vi "ATEQread气密机一.vi"(7 "baud rate (9600)":u32=57600 caption="波特率(9600)", 8 "VISA resource name":refnum<visa-resource-name>="COM3" caption="COM", 9 "从站地址":u8=2 format="%x", 10 "Read Address":u16 format="%x", 11 "The number of Read":u32) -> (0 "Read Values":string, 1 "ReturnResultValues":u16[](array[numeric]), 2 "Read Status":bool)   [LabVIEW 2014]
uses:
  <vilib>/Instr/_visa.llb/VISA Configure Serial Port (Instr).vi
panel:
  out "Serial Settings:Number of Bytes at Serial Port":u32
  out "Result":string
  out "Read Return Value":string
  out "Send Read Date":string
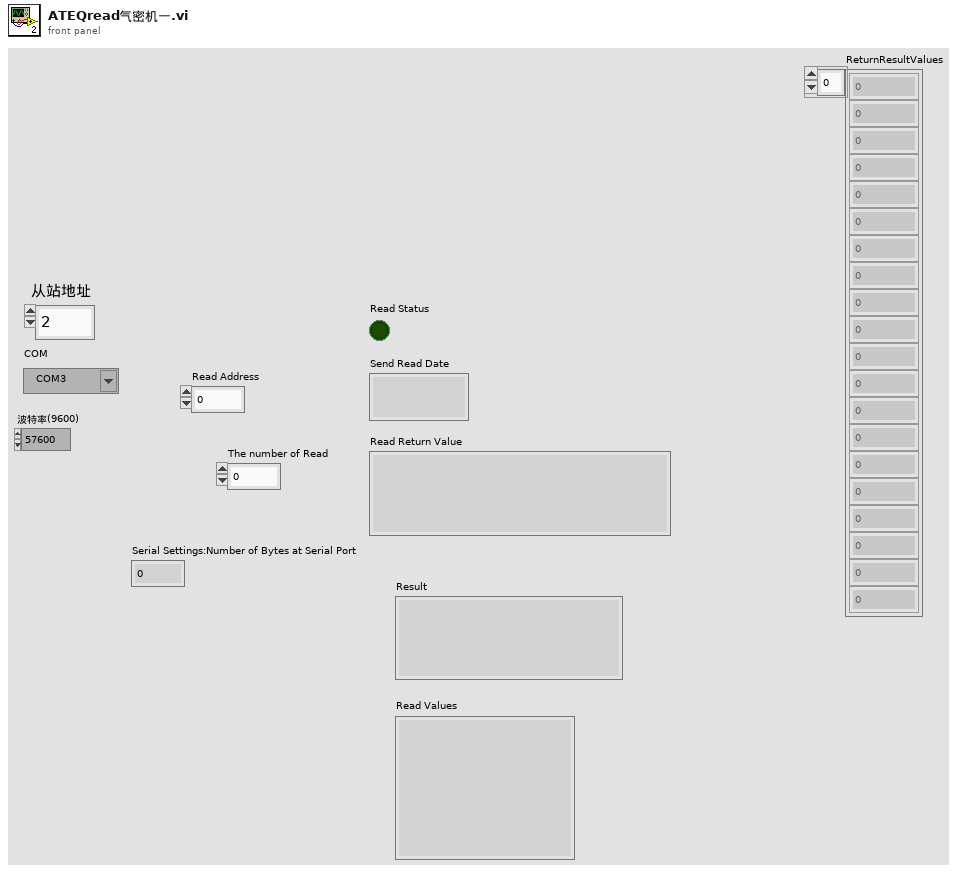
[diagram p1: front panel]
types:
  T1 = enum16{"big-endian, network order", "native, host order", "little-endian"}
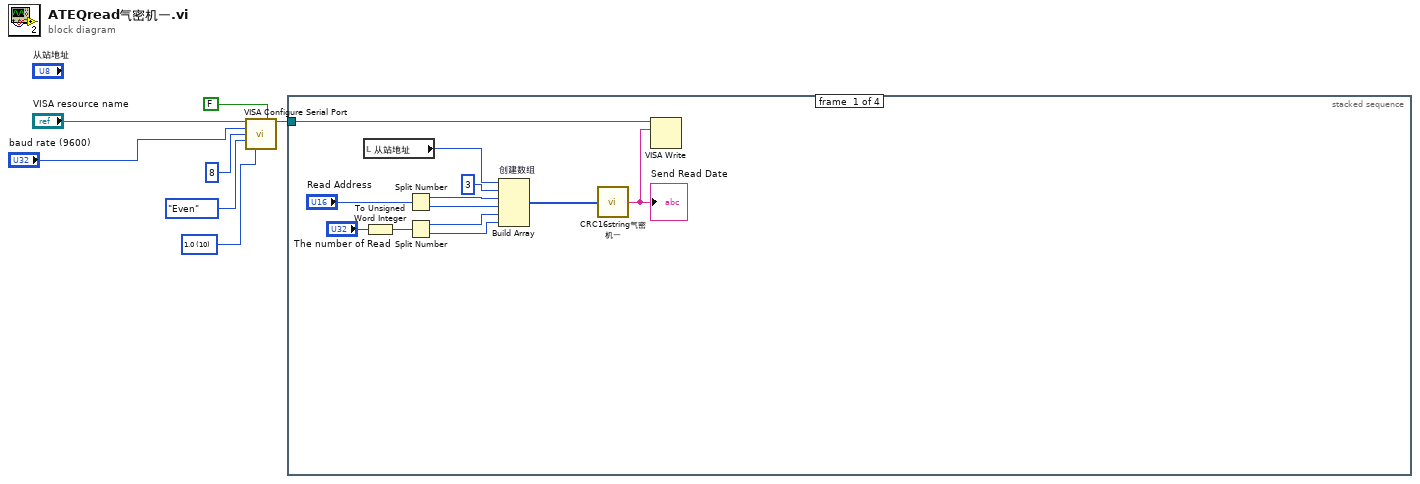
[diagram p0: block diagram]
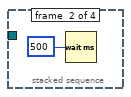
[diagram p2: hidden frame]
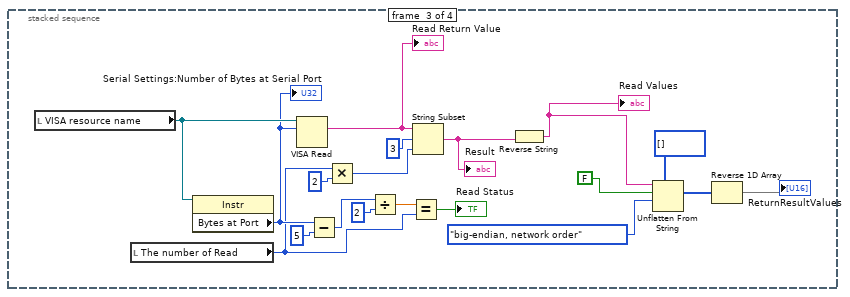
[diagram p3: hidden frame]
diagram:
  w7 = u16 10 items=["1.0"=10, "1.5"=15, "2.0"=20] ("stop bits (10: 1 bit)")
  n1 = call-poly "VISA Configure Serial Port"("VISA resource name"="VISA resource name", "Enable Termination\nChar (T)"=FALSE ("Enable Termination\nChar (T)"), "baud rate (9600)"="baud rate (9600)", "data bits (8)"=u16 8, "parity (0:none)"=enum16{"None", "Odd", "Even", "Mark", "Space"}."Even", "stop bits (10: 1 bit)"=w7) -> ("VISA resource name out"=w2:refnum<visa-resource-name>)  [unwired: 8 in, 1 out]
  n2 = stacked-sequence {
    tunnel: w2 -> [w8 _ _ _]
    frame #0 {
      n3 = local read "从站地址"() -> (w9:u8)
      n4 = To Unsigned Word Integer(number="The number of Read") -> (unsigned 16bit integer=w17:u16)
      n5 = Split Number(x="Read Address") -> (hi(x)=w15:u8, lo(x)=w14:u8)
      n6 = Split Number(x=w17) -> (hi(x)=w10:u8, lo(x)=w13:u8)
      n7 = Build Array "创建数组"(w9, u8 3, w15, w14, w10, w13) -> (w12:u8[])
      n8 = call "CRC16string气密机一.vi"("数组"=w12) -> ("要发送的数据"=w11:string)
      "Send Read Date" <- w11
      n9 = VISA Write(VISA resource name=w8, write buffer=w11) -> ()  [unwired: 1 in, 3 out]
    }
    frame #1 {
      n10 = Wait (ms)(milliseconds to wait=u32 500 ("等待时间（毫秒）")) -> ()  [unwired: 1 out]
    }
    frame #2 {
      n11 = local read "VISA resource name"() -> (w39:refnum<visa-resource-name>)
      n12 = local read "The number of Read"() -> (w32:u32)
      n13 = property class="Instr"(reference=w39) -> ("Bytes at Port"=w38:u32)  [unwired: 1 in, 2 out]
      "Serial Settings:Number of Bytes at Serial Port" <- w38
      n14 = VISA Read(VISA resource name=w39, byte count=w38) -> (read buffer=w34:string)  [unwired: 1 in, 3 out]
      "Read Return Value" <- w34
      n15 = Subtract(x=w38, y=5) -> (x-y=w28:u32)
      n16 = Multiply(x=w32, y=u32 2) -> (x*y=w30:u32)
      n17 = Divide(x=w28, y=2) -> (x/y=w35:dbl)
      n18 = Equal?(x=w35, y=w32) -> (x = y?=→"Read Status":bool)
      n19 = String Subset(string=w34, offset (0)=3 ("偏移量(0)"), length (rest)=w30) -> (substring=w27:string)
      "Result" <- w27
      n20 = Reverse String(1:w27) -> (0:w22:string)
      "Read Values" <- w22
      n21 = Unflatten From String(type=u16[] [] ("初始化的数组"), binary string=w22, data includes array or string size? (T)=FALSE ("数据中包含数组或字符串大小？(T)"), byte order (0:big-endian, network order)=T1."big-endian, network order" ("字节顺序(0:big-endian, network order)")) -> (value=w23:u16[])  [unwired: 1 in, 2 out]
      n22 = Reverse 1D Array(array=w23) -> (reversed array=→"ReturnResultValues":u16[])
    }
    frame #3 {
    }
  }
